vi "RT Host Test.vi"() -> ()   [LabVIEW 2015]
uses:
  <vilib>/FPGAPlugInAG/PXI-7953R/niLvFpga_Open_PXI-7953R.vi
  <vilib>/rvi/interface/common/dynamic/niFpgaDynamicAddResources.vi
  <vilib>/FPGAPlugInAG/Dynamic/niLvFpga_Reset_Dynamic.vi
  <vilib>/rvi/interface/common/niFpgaWaitOnOcc.vi
  <vilib>/Utility/error.llb/Error Cluster From Error Code.vi
  <vilib>/rvi/errors/niLvFpgaAdjustHostInterfaceError.vi
  <vilib>/FPGAPlugInAG/Dynamic/niLvFpga_Run_Dynamic.vi
  <vilib>/RVI Host/nirviSupport.llb/nirviErrorClusterFromErrorCode.vi
  <vilib>/FPGAPlugInAG/Dynamic/niLvFpga_Close_Dynamic.vi
  <vilib>/rvi/interface/nirviOpenFPGA/nirviOpenFPGA.xnode
  FPGA Bitfiles/7953_FPGA VI_Simulated.lvbitx
  <vilib>/rvi/interface/nirviMethod/nirviMethod.xnode
  <vilib>/rvi/interface/nirviReadWriteControl/nirviReadWriteControl.xnode
  <vilib>/rvi/interface/nirviCloseFPGA/nirviCloseFPGA.xnode
  <vilib>/FPGAPlugInAG/Dynamic/niLvFpga_ConfigureFifo_Dynamic.vi
  <vilib>/rvi/errors/niLvFpgaMergeErrorWithErrorCode.vi
  <vilib>/FPGAPlugInAG/Dynamic/niLvFpga_StartFifo_Dynamic.vi
  NiFpgaLv.dll
  <vilib>/rvi/interface/Simulation/niFpgaSimulationCallBeginRW.vi
  <vilib>/rvi/interface/nirviMethod/StockFPGA_InlinedMethodWaitForSingleIRQ.vi
  <vilib>/FPGAPlugInAG/Dynamic/niLvFpga_WaitOnIrq_Dynamic.vi
  <vilib>/FPGAPlugInAG/Dynamic/niLvFpga_AcknowledgeIrq_Dynamic.vi
  <vilib>/FPGAPlugInAG/Dynamic/niLvFpga_ReadFifo_Dynamic.vi
panel:
  out "Intermediate FIFO Write Timeout":bool
  out "Acqusition Loop Ticks":u32
  out "Host DMA Out?":bool
  out "Intermediate Time Out?":bool
  out "error out":errorcluster
  out "Injector Samples":dbl
  out "Injector Period":dbl
  out "Injector Index":dbl
  in  "stop":bool
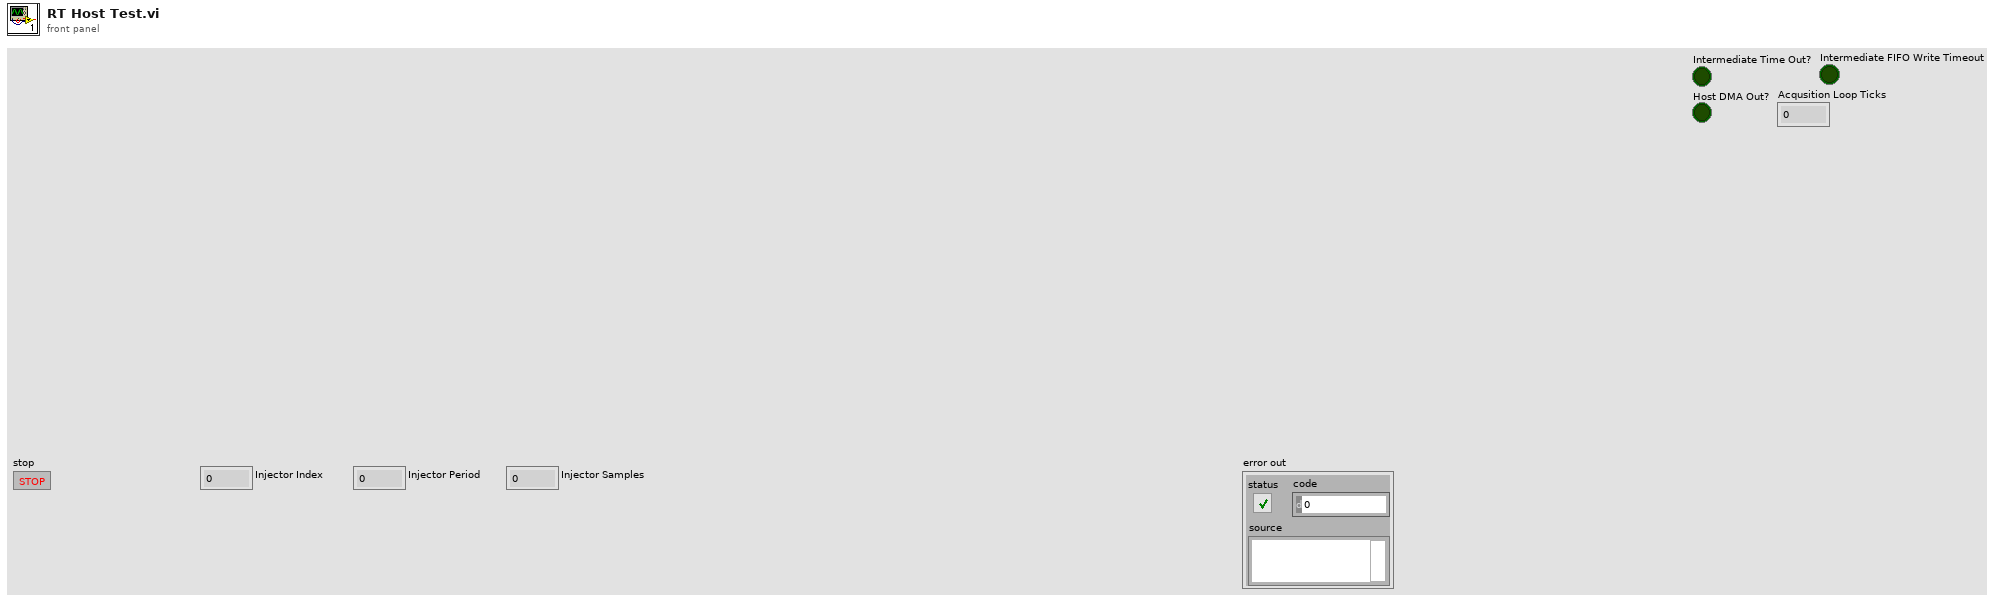
[diagram p1: front panel]
types:
  T1 = cluster{"Enable?":bool, "Initial Voltage Threshold":fxp<+/-,32,8>, "Event Dwell Limit":u16, "Voltage Gain":fxp<+/-,32,8>, "Current Gain":fxp<+/-,32,8>}
  T2 = cluster{"Voltage Offset":fxp<+/-,32,8>, "Current Offset":fxp<+/-,32,8>}
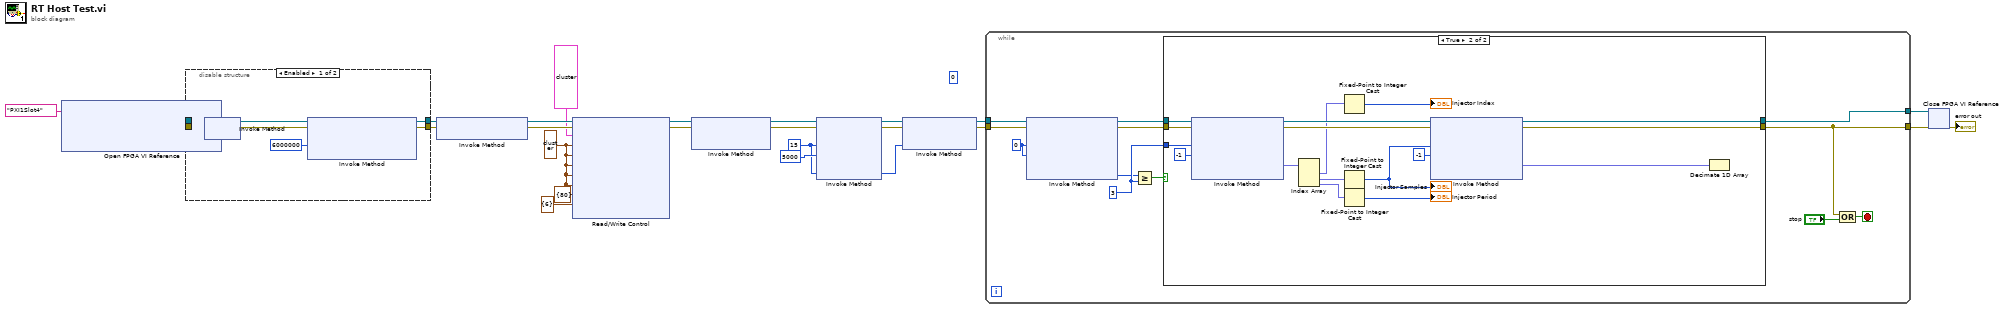
[diagram p0: block diagram]
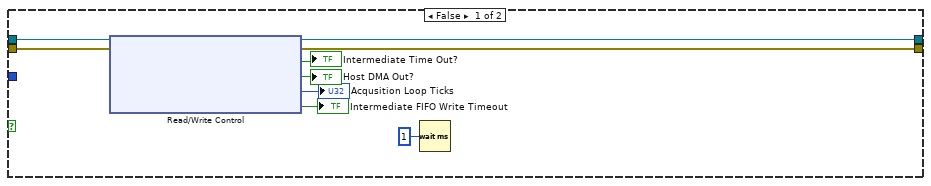
[diagram p2: hidden frame]
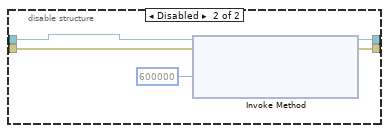
[diagram p3: hidden frame]
diagram:
  (unwired) 0
  w9 = T2 {"Voltage Offset"=0.0, "Current Offset"=0.0} ("Settings.Index0.Injector0")
  w13 = 15 ("IRQ Number(s)")
  n1 = xnode "Open FPGA VI Reference"("resource name"=tag "PXI1Slot4") -> ("FPGA VI Reference Out"=w4:refnum<k20>, "error out"=w5:errorcluster)  [unwired: 1 in]
  n2 = disable-structure shown="Enabled" {
    disable-tunnel: [w30 w35] -> w24
    disable-tunnel: [w29 w34] -> w23
    disable-tunnel: w5 -> [w28 w33]
    disable-tunnel: w4 -> [w26 w32]
    frame Enabled {
      n3 = xnode "Invoke Method"("FPGA VI Reference In"=w26, "error in"=w28) -> ("FPGA VI Reference Out"=w25:refnum<k20>, "error out"=w27:errorcluster)
      n4 = xnode "Invoke Method"("FPGA VI Reference In"=w25, "error in"=w27, "Requested Depth"=6000000) -> ("FPGA VI Reference Out"=w30:refnum<k20>, "error out"=w29:errorcluster)  [unwired: 1 out]
    }
    frame Disabled {
      n5 = xnode "Invoke Method"("FPGA VI Reference In"=w32, "error in"=w33, "Requested Depth"=600000) -> ("FPGA VI Reference Out"=w35:refnum<k20>, "error out"=w34:errorcluster)  [unwired: 1 out]
    }
  }
  n6 = xnode "Invoke Method"("FPGA VI Reference In"=w24, "error in"=w23) -> ("FPGA VI Reference Out"=w22:refnum<k20>, "error out"=w21:errorcluster)
  n7 = xnode "Read/Write Control"("FPGA VI Reference In"=w22, "error in"=w21, "Settings.Global"=T1 {"Enable?"=TRUE, "Initial Voltage Threshold"=6.0, "Event Dwell Limit"=1500, "Voltage Gain"=1.0, "Current Gain"=1.0}, "Settings.Index0.Injector0"=w9, "Settings.Index1.Injector1"=w9, "Settings.Index2.Injector2"=w9, "Settings.Index3.Injector3"=w9, "Settings.Index4.Injector4"=w9, "Settings.Index5.Injector5"=w9, "Settings.Timing"=cluster{"Injector Sample Period (Ticks)":u32} {"Injector Sample Period (Ticks)"=80}, "Settings.DMA"=cluster{"# of Injectors":u8} {"# of Injectors"=6}) -> ("FPGA VI Reference Out"=w20:refnum<k20>, "error out"=w19:errorcluster)
  n8 = xnode "Invoke Method"("FPGA VI Reference In"=w20, "error in"=w19) -> ("FPGA VI Reference Out"=w18:refnum<k20>, "error out"=w17:errorcluster)  [unwired: 1 in]
  n9 = xnode "Invoke Method"("FPGA VI Reference In"=w18, "error in"=w17, "IRQ Number(s)"=w13, "Timeout (ms)"=5000) -> ("FPGA VI Reference Out"=w15:refnum<k20>, "error out"=w14:errorcluster)  [unwired: 2 out]
  n10 = xnode "Invoke Method"("FPGA VI Reference In"=w15, "error in"=w14, "IRQ Number(s)"=w13) -> ("FPGA VI Reference Out"=w12:refnum<k20>, "error out"=w11:errorcluster)
  n11 = while {
    tunnel: w12 -> [w37]
    tunnel: w11 -> [w38]
    tunnel: [w43] -> w7
    tunnel: [w42] -> w6
    stop <- w44 stop-if-true
    w41 = u32 3 ("y")
    w40 = u32 0 ("Requested Depth")
    n12 = xnode "Invoke Method"("FPGA VI Reference In"=w37, "error in"=w38, "Number of Elements"=w40, "Timeout (ms)"=w40) -> ("FPGA VI Reference Out"=w48:refnum<k20>, "error out"=w47:errorcluster, "Elements Remaining"=w39:u32)  [unwired: 1 out]
    n13 = Greater Or Equal?(x=w39, y=w41) -> (x >= y?=w46:bool)
    n14 = case shown="True" w46 {
      tunnel: w48 -> [w52 w74]
      tunnel: w47 -> [w51 w73]
      tunnel: [w50 w69] -> w43
      tunnel: [w49 w67] -> w42
      tunnel: w41 -> [_ w71]
      frame False {
        n15 = xnode "Read/Write Control"("FPGA VI Reference In"=w52, "error in"=w51) -> ("FPGA VI Reference Out"=w49:refnum<k20>, "error out"=w50:errorcluster, "Intermediate Time Out?"=→"Intermediate Time Out?":bool, "Host DMA Out?"=→"Host DMA Out?":bool, "Acqusition Loop Ticks"=→"Acqusition Loop Ticks":u32, "Intermediate FIFO Write Timeout"=→"Intermediate FIFO Write Timeout":bool)
        n16 = Wait (ms)(milliseconds to wait=u32 1) -> ()  [unwired: 1 out]
      }
      frame True {
        n17 = xnode "Invoke Method"("FPGA VI Reference In"=w74, "error in"=w73, "Number of Elements"=w71, "Timeout (ms)"=-1) -> ("FPGA VI Reference Out"=w68:refnum<k20>, "error out"=w70:errorcluster, "Data"=w66:fxp<+/-,32,8>[])  [unwired: 1 out]
        n18 = Index Array(array=w66) -> (element #1=w64:fxp<+/-,32,8>, element #2=w62:fxp<+/-,32,8>, element #3=w61:fxp<+/-,32,8>)  [unwired: 3 in]
        n19 = Fixed-Point to Integer Cast(1:w64) -> (0:→"Injector Index":i32)
        n20 = Fixed-Point to Integer Cast(1:w62) -> (0:w59:i32)
        "Injector Samples" <- w59
        n21 = Fixed-Point to Integer Cast(1:w61) -> (0:→"Injector Period":i32)
        n22 = xnode "Invoke Method"("FPGA VI Reference In"=w68, "error in"=w70, "Number of Elements"=w59, "Timeout (ms)"=-1) -> ("FPGA VI Reference Out"=w67:refnum<k20>, "error out"=w69:errorcluster, "Data"=w58:fxp<+/-,32,8>[])  [unwired: 1 out]
        n23 = Decimate 1D Array(w58) -> ()  [unwired: 2 out]
      }
    }
    n24 = Compound Arithmetic op=OR(w43, "stop") -> (w44:bool)
  }
  n25 = xnode "Close FPGA VI Reference"("FPGA VI Reference In"=w6, "error in"=w7) -> ("error out"=→"error out":errorcluster)
